vi "AWG Calculate Wave Ampl.vi"(8 "Offset":dbl, 9 "Gain":dbl, 11 "Amplitude":dbl) -> (3 "Waveform Amplitude":dbl)   [LabVIEW 2013]
panel:
  in  "AmpGain":dbl=15.0
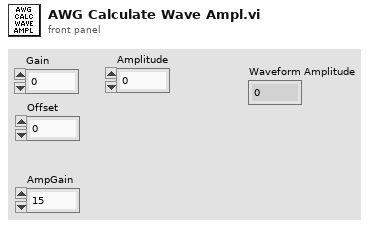
[diagram p1: front panel]
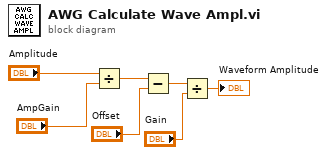
[diagram p0: block diagram]
diagram:
  n1 = Divide(x="Amplitude", y="AmpGain") -> (x/y=w1:dbl)
  n2 = Subtract(x=w1, y="Offset") -> (x-y=w7:dbl)
  n3 = Divide(x=w7, y="Gain") -> (x/y=→"Waveform Amplitude":dbl)
